vi "Interpolate 4 Arrays BY DP.vi"(0 "HP Higher DP Array":dbl[](array[numeric])=[65.37068268, 76.39538331, 13.47092917, 29.94278114, 60.23898441], 1 "Pressure Z":dbl=0.9850456142413025, 2 "RH Z":dbl=0.75, 5 "HP Lower DP Array":dbl[](array[numeric])=[62.63251626, 63.47717435, 13.43164845, 27.92329599, 55.18152622], 9 "LP Higher DP Array":dbl[](array[numeric])=[65.31206979, 77.81069741, 13.72049378, 30.16403517, 60.23898441], 11 "LP Lower DP Array":dbl[](array[numeric])=[62.55302827, 64.64967087, 13.67974634, 28.10659069, 55.18152622], 12 "1st Known Index":u16(ring) items=["DB", "WB", "RH", "HR", "Gr", "Vol", "h", "Dp"]) -> (8 "Output Array":dbl[](array[numeric]))   [LabVIEW 2020]
panel:
  out "Out 5":dbl
  out "Out 4":dbl
  out "Out 3":dbl
  out "Out 2":dbl
  out "Out 1":dbl
  out "Out 0":dbl
  # "DB = 0\nWB = 1\nRH = 2\nHR = 3\nGr = 4\nVol = 5\nh = 6\nDp = 7"
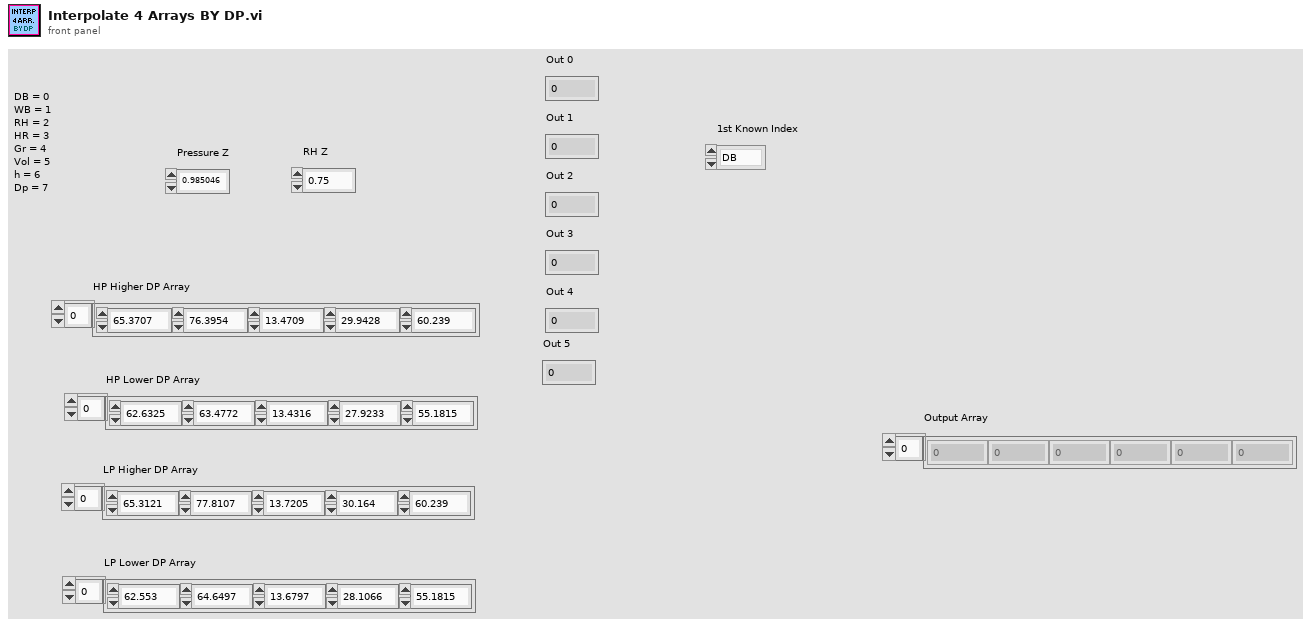
[diagram p1: front panel]
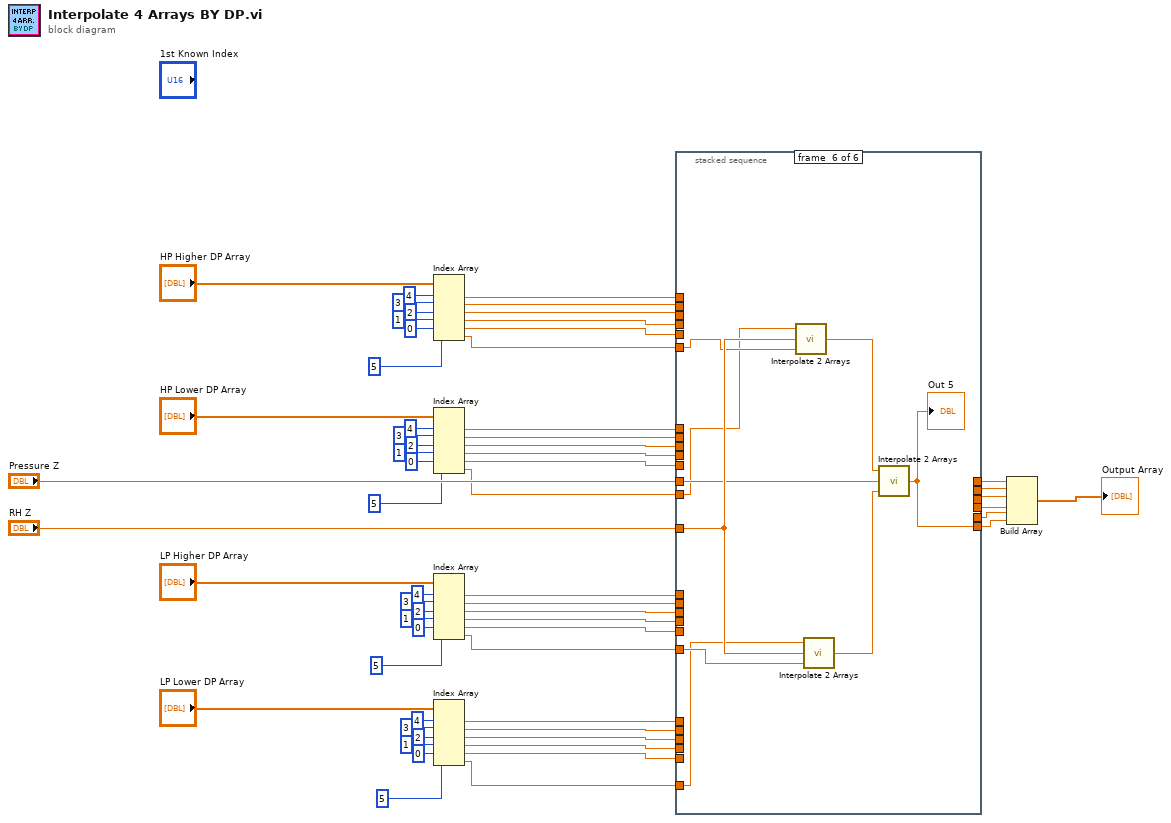
[diagram p0: block diagram]
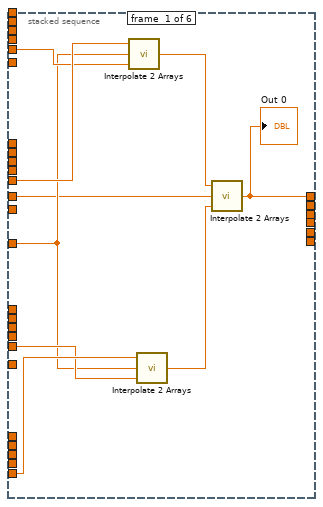
[diagram p2: hidden frame]
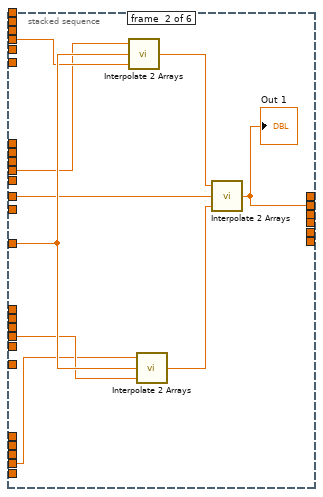
[diagram p3: hidden frame]
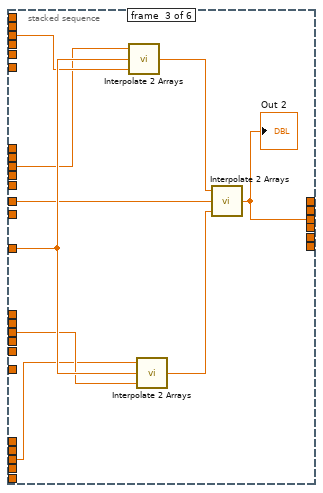
[diagram p4: hidden frame]
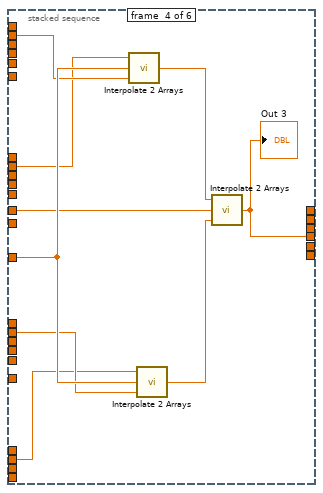
[diagram p5: hidden frame]
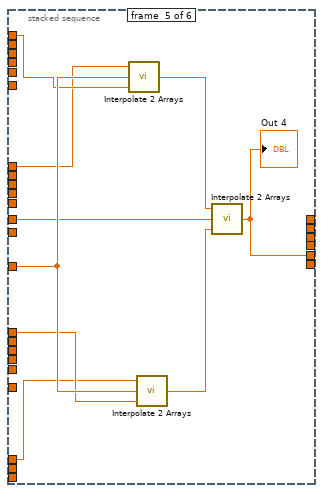
[diagram p6: hidden frame]
diagram:
  n1 = Index Array(array="HP Higher DP Array", index #1=4 ("index"), index #2=3 ("index"), index #3=2 ("index"), index #4=1 ("index"), index #5=0 ("index"), index #6=5 ("index")) -> (element #1=w37:dbl, element #2=w36:dbl, element #3=w35:dbl, element #4=w34:dbl, element #5=w33:dbl, element #6=w4:dbl)
  n2 = Index Array(array="HP Lower DP Array", index #1=4 ("index"), index #2=3 ("index"), index #3=2 ("index"), index #4=1 ("index"), index #5=0 ("index"), index #6=5 ("index")) -> (element #1=w32:dbl, element #2=w31:dbl, element #3=w30:dbl, element #4=w29:dbl, element #5=w28:dbl, element #6=w3:dbl)
  n3 = Index Array(array="LP Higher DP Array", index #1=4 ("index"), index #2=3 ("index"), index #3=2 ("index"), index #4=1 ("index"), index #5=0 ("index"), index #6=5 ("index")) -> (element #1=w27:dbl, element #2=w26:dbl, element #3=w25:dbl, element #4=w24:dbl, element #5=w23:dbl, element #6=w2:dbl)
  n4 = Index Array(array="LP Lower DP Array", index #1=4 ("index"), index #2=3 ("index"), index #3=2 ("index"), index #4=1 ("index"), index #5=0 ("index"), index #6=5 ("index")) -> (element #1=w22:dbl, element #2=w21:dbl, element #3=w20:dbl, element #4=w19:dbl, element #5=w18:dbl, element #6=w1:dbl)
  n5 = stacked-sequence {
    tunnel: w37 -> [_ _ _ _ w101 _]
    tunnel: w36 -> [_ _ _ w92 _ _]
    tunnel: w35 -> [_ _ w83 _ _ _]
    tunnel: w34 -> [_ w74 _ _ _ _]
    tunnel: w33 -> [w69 _ _ _ _ _]
    tunnel: "Pressure Z" -> [w63 w76 w85 w94 w103 w112]
    tunnel: "RH Z" -> [w66 w79 w88 w97 w106 w115]
    tunnel: w32 -> [_ _ _ _ w100 _]
    tunnel: w31 -> [_ _ _ w91 _ _]
    tunnel: w30 -> [_ _ w82 _ _ _]
    tunnel: w29 -> [_ w73 _ _ _ _]
    tunnel: w28 -> [w70 _ _ _ _ _]
    tunnel: w27 -> [_ _ _ _ w99 _]
    tunnel: w26 -> [_ _ _ w90 _ _]
    tunnel: w25 -> [_ _ w81 _ _ _]
    tunnel: w24 -> [_ w72 _ _ _ _]
    tunnel: w23 -> [w67 _ _ _ _ _]
    tunnel: w22 -> [_ _ _ _ w98 _]
    tunnel: w21 -> [_ _ _ w89 _ _]
    tunnel: w20 -> [_ _ w80 _ _ _]
    tunnel: w19 -> [_ w71 _ _ _ _]
    tunnel: w18 -> [w68 _ _ _ _ _]
    tunnel: [w62 _ _ _ _ _] -> w15
    tunnel: [_ w75 _ _ _ _] -> w13
    tunnel: [_ _ w84 _ _ _] -> w12
    tunnel: [_ _ _ w93 _ _] -> w11
    tunnel: [_ _ _ _ w102 _] -> w10
    tunnel: [_ _ _ _ _ w111] -> w5
    tunnel: w4 -> [_ _ _ _ _ w110]
    tunnel: w3 -> [_ _ _ _ _ w109]
    tunnel: w2 -> [_ _ _ _ _ w108]
    tunnel: w1 -> [_ _ _ _ _ w107]
    frame #0 {
      n6 = call "Interpolate 2 Arrays.vi"("Y2"=w69, "Z"=w66, "Y1"=w70) -> ("Yi"=w65:dbl)
      n7 = call "Interpolate 2 Arrays.vi"("Y2"=w67, "Z"=w66, "Y1"=w68) -> ("Yi"=w64:dbl)
      n8 = call "Interpolate 2 Arrays.vi"("Y2"=w64, "Z"=w63, "Y1"=w65) -> ("Yi"=w62:dbl)
      "Out 0" <- w62
    }
    frame #1 {
      n9 = call "Interpolate 2 Arrays.vi"("Y2"=w74, "Z"=w79, "Y1"=w73) -> ("Yi"=w78:dbl)
      n10 = call "Interpolate 2 Arrays.vi"("Y2"=w72, "Z"=w79, "Y1"=w71) -> ("Yi"=w77:dbl)
      n11 = call "Interpolate 2 Arrays.vi"("Y2"=w77, "Z"=w76, "Y1"=w78) -> ("Yi"=w75:dbl)
      "Out 1" <- w75
    }
    frame #2 {
      n12 = call "Interpolate 2 Arrays.vi"("Y2"=w83, "Z"=w88, "Y1"=w82) -> ("Yi"=w87:dbl)
      n13 = call "Interpolate 2 Arrays.vi"("Y2"=w81, "Z"=w88, "Y1"=w80) -> ("Yi"=w86:dbl)
      n14 = call "Interpolate 2 Arrays.vi"("Y2"=w86, "Z"=w85, "Y1"=w87) -> ("Yi"=w84:dbl)
      "Out 2" <- w84
    }
    frame #3 {
      n15 = call "Interpolate 2 Arrays.vi"("Y2"=w92, "Z"=w97, "Y1"=w91) -> ("Yi"=w96:dbl)
      n16 = call "Interpolate 2 Arrays.vi"("Y2"=w90, "Z"=w97, "Y1"=w89) -> ("Yi"=w95:dbl)
      n17 = call "Interpolate 2 Arrays.vi"("Y2"=w95, "Z"=w94, "Y1"=w96) -> ("Yi"=w93:dbl)
      "Out 3" <- w93
    }
    frame #4 {
      n18 = call "Interpolate 2 Arrays.vi"("Y2"=w101, "Z"=w106, "Y1"=w100) -> ("Yi"=w105:dbl)
      n19 = call "Interpolate 2 Arrays.vi"("Y2"=w99, "Z"=w106, "Y1"=w98) -> ("Yi"=w104:dbl)
      n20 = call "Interpolate 2 Arrays.vi"("Y2"=w104, "Z"=w103, "Y1"=w105) -> ("Yi"=w102:dbl)
      "Out 4" <- w102
    }
    frame #5 {
      n21 = call "Interpolate 2 Arrays.vi"("Y2"=w110, "Z"=w115, "Y1"=w109) -> ("Yi"=w114:dbl)
      n22 = call "Interpolate 2 Arrays.vi"("Y2"=w108, "Z"=w115, "Y1"=w107) -> ("Yi"=w113:dbl)
      n23 = call "Interpolate 2 Arrays.vi"("Y2"=w113, "Z"=w112, "Y1"=w114) -> ("Yi"=w111:dbl)
      "Out 5" <- w111
    }
  }
  n24 = Build Array(w15, w13, w12, w11, w10, w5) -> (→"Output Array":dbl[])
